vi "Max ODBC Driver Version.vi"(10 "Drivers":string[](array[string])) -> (2 "driver":string)   [LabVIEW 2018]
panel:
  out "Driver Version":dbl[](array[numeric])
  out "MySQL Drivers":string[](array[string])
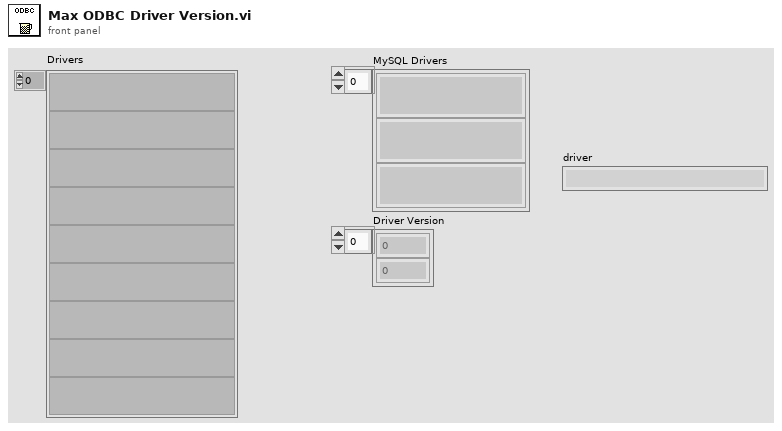
[diagram p1: front panel]
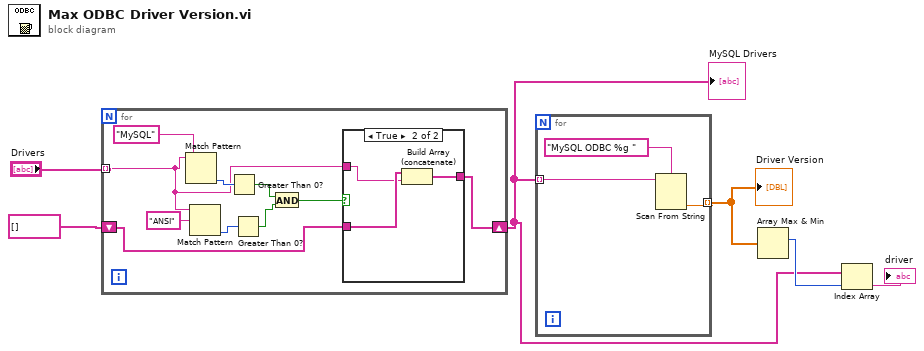
[diagram p0: block diagram]
diagram:
  n1 = for {
    tunnel: "Drivers" -> [w8] mode=indexing
    shift-right: [w7] -> w2
    shift-left: string[] [] -> [w9]
    n2 = Match Pattern(string=w8, regular expression="MySQL") -> (offset past match=w14:i32)  [unwired: 1 in, 3 out]
    n3 = Match Pattern(string=w8, regular expression="ANSI") -> (offset past match=w13:i32)  [unwired: 1 in, 3 out]
    n4 = Greater Than 0?(x=w14) -> (x > 0?=w12:bool)
    n5 = Greater Than 0?(x=w13) -> (x > 0?=w11:bool)
    n6 = And(x=w12, y=w11) -> (x .and. y?=w10:bool)
    n7 = case shown="True" w10 {
      tunnel: w9 -> [w17 w20]
      tunnel: w8 -> [_ w19]
      tunnel: [w17 w18] -> w7
      frame False {
      }
      frame True {
        n8 = Build Array (concatenate)(w20, w19) -> (w18:string[])
      }
    }
  }
  "MySQL Drivers" <- w2
  n9 = for {
    tunnel: w2 -> [w23] mode=indexing
    tunnel: [w21] -> w4 mode=indexing
    n10 = Scan From String(format string="MySQL ODBC %g ", input string=w23) -> (output 1=w21:dbl)  [unwired: 3 in, 3 out]
  }
  "Driver Version" <- w4
  n11 = Array Max & Min(array=w4) -> (max index (indices)=w3:i32)  [unwired: 3 out]
  n12 = Index Array(array=w2, index=w3) -> (element=→"driver":string)
